vi "Get Geometric Mean Anomaly.vi"(11 "Julian Century":dbl) -> (3 "Mean Anomaly":dbl)   [LabVIEW 2014, in "Solar Calculations.lvlib"]
doc: "Calculates the geometric mean anomaly of the sun and returns it in degrees."
uses:
  Solar Calculations.lvlib
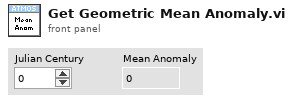
[diagram p1: front panel]
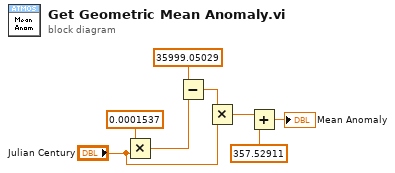
[diagram p0: block diagram]
diagram:
  n1 = Multiply(x=0.0001537, y="Julian Century") -> (x*y=w2:dbl)
  n2 = Subtract(x=35999.05029, y=w2) -> (x-y=w4:dbl)
  n3 = Multiply(x=w4, y="Julian Century") -> (x*y=w6:dbl)
  n4 = Add(x=w6, y=357.52911) -> (x+y=→"Mean Anomaly":dbl)
